vi "Update Values.vi"(8 "error in (no error)":errorcluster, 11 "TelemetryDebug in":refnum<class "TelemetryDebug.lvclass">) -> (0 "error out":errorcluster, 3 "TelemetryDebug out":refnum<class "TelemetryDebug.lvclass">)   [LabVIEW 2020, in "VectoTools.lvlib" / "TelemetryDebug.lvclass"]
uses:
  TelemetryDebug.lvclass
  Tree Entry.ctl
  TelemetryDebug.lvclass/TelemetryDebug.ctl
  Vecto/Group/Group.lvclass/Group.ctl
  Vecto/Group/Group.lvclass
  Vecto/DiscoveryService/DiscoveryService.lvclass
  Vecto/ChannelService/ChannelService.lvclass
  Vecto/Group Config/Group Config.lvclass
  Vecto/Channel Config/Channel Config.lvclass
panel:
  in  "Numeric":dbl format="%<%Y-%m-%dT%H:%M:%S%3u\n>T"
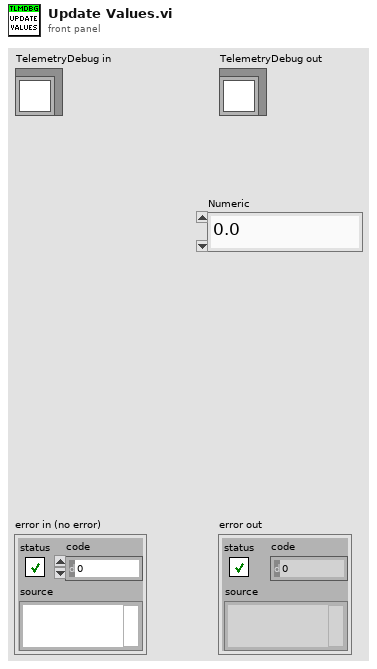
[diagram p1: front panel]
types:
  T1 = typedef "VectoTools.lvlib/TelemetryDebug.lvclass/Tree Entry.ctl" = cluster{"Hierarchy":string[], "Name":string, "Columns":string[]}
  T2 = typedef "Discovery.lvlib/Data.ctl" = cluster{"node_id":u32, "name":string, "ip":u32, "status":string, "services":T3[], "capabilities":string[], "system":string, "cluster":string, "app_version":string, "cfg_version":string}
  T3 = typedef "Service.lvlib/Data.ctl" = cluster{"type":T4, "port":i32}
  T4 = typedef "ServiceType.lvlib/Enumeration.ctl" = enum16{"SERVICETYPE_UNKNOWN", "SERVICETYPE_TCPSERVER", "SERVICETYPE_HTTPSERVER"}
  T5 = typedef "LVNodeAndColumnTypeDef.ctl" = cluster{"Node":string, "Column":i32}
  T6 = typedef "VectoConfig.lvlib/Group Info.ctl" = cluster{"System":string, "Cluster":string, "Node":string, "Task":string, "Name":string}
  T7 = typedef "VectoConfig.lvlib/Channel Info.ctl" = cluster{"Name":string, "Group":string, "Owning Node":string, "Owning Task":string, "Resource":string}
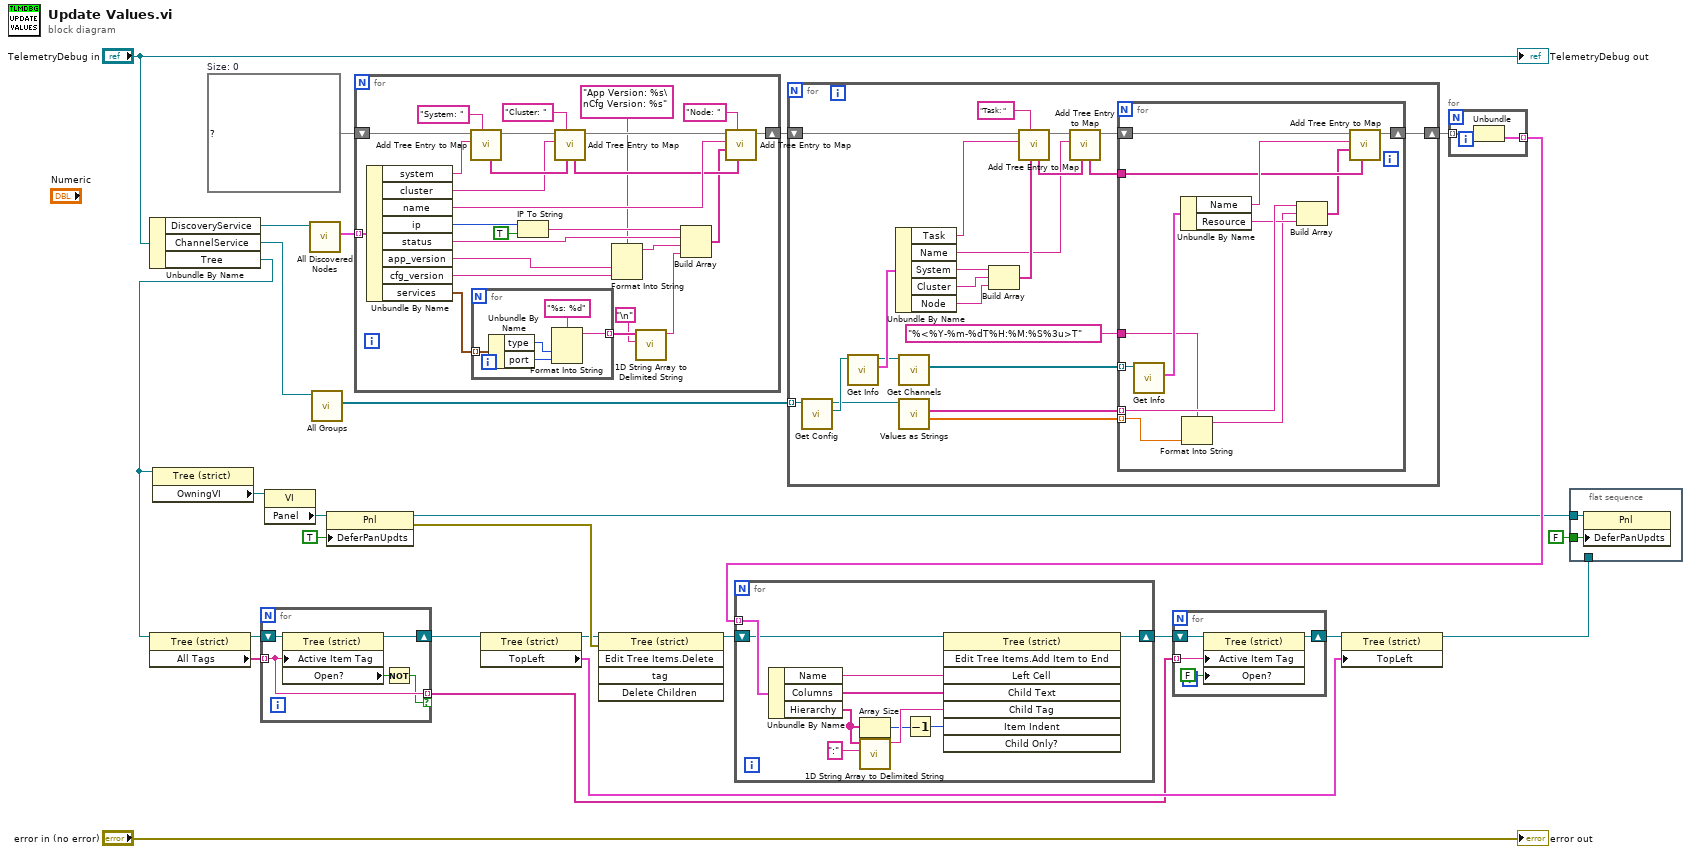
[diagram p0: block diagram]
diagram:
  w22 = map{string[], T1} {}  # Size: 0
  n1 = Unbundle By Name("TelemetryDebug in") -> ("DiscoveryService"=w24:refnum<class "DiscoveryService.lvclass">, "ChannelService"=w14:refnum<class "ChannelService.lvclass">, "Tree"=w1:refnum<vi>)
  n2 = property class="Tree (strict)"(reference=w1) -> (reference out=w7:refnum<vi>, "All Tags"=w8:string[])  [unwired: 1 in, 1 out]
  n3 = property class="Tree (strict)"(reference=w1) -> ("OwningVI"=w19:refnum<vi>)  [unwired: 1 in, 2 out]
  n4 = for {
    tunnel: w8 -> [w30] mode=indexing
    shift-right: [w28] -> w6
    shift-left: w7 -> [w32]
    tunnel: [w30] -> w5 mode=indexing if=w29
    n5 = property class="Tree (strict)"(reference=w32, "Active Item Tag"=w30) -> (reference out=w28:refnum<vi>, "Open?"=w31:bool)  [unwired: 1 in, 1 out]
    n6 = Not(x=w31) -> (.not. x?=w29:bool)
  }
  n7 = property class="VI"(reference=w19) -> ("Panel"=w18:refnum<vi>)  [unwired: 1 in, 2 out]
  n8 = call "All Discovered Nodes.vi"("DiscoveryService in"=w24) -> ("Nodes"=w23:T2[])  [unwired: 8 in, 2 out]
  n9 = call "All Groups.vi"("ChannelService in"=w14) -> ("Groups"=w11:refnum<class "Group.lvclass">[])  [unwired: 8 in, 2 out]
  n10 = property class="Pnl"(reference=w18, "DeferPanUpdts"=TRUE ("Defer Panel Updates")) -> (reference out=w15:refnum<vi>, error out=w27:errorcluster)  [unwired: 1 in]
  n11 = for {
    tunnel: w23 -> [w58] mode=indexing
    shift-right: [w49] -> w13
    shift-left: w22 -> [w57]
    n12 = Unbundle By Name(w58) -> ("system"=w56:string, "cluster"=w53:string, "name"=w51:string, "ip"=w48:u32, "status"=w44:string, "app_version"=w36:string, "cfg_version"=w35:string, "services"=w46:T3[])
    n13 = call "Add Tree Entry to Map.vi"("Name Prefix (none)"="System: ", "Name"=w56, "Map in"=w57) -> ("Map"=w54:map{string[], T1}, "Hierarchy"=w55:string[])  [unwired: 7 in]
    n14 = for {
      tunnel: w46 -> [w63] mode=indexing
      tunnel: [w59] -> w39 mode=indexing
      n15 = Unbundle By Name(w63) -> ("type"=w61:T4, "port"=w60:i32)
      n16 = Format Into String(format string="%s: %d", w61, w60) -> (resulting string=w59:string)  [unwired: 2 in, 1 out]
    }
    n17 = IP To String(1:TRUE ("dot notation? (F)"), 2:w48) -> (0:w45:string)
    n18 = call "Add Tree Entry to Map.vi"("Parent (None)"=w55, "Name Prefix (none)"="Cluster: ", "Name"=w53, "Map in"=w54) -> ("Map"=w52:map{string[], T1}, "Hierarchy"=w50:string[])  [unwired: 6 in]
    n19 = Format Into String(format string="App Version: %s\nCfg Version: %s", w36, w35) -> (resulting string=w33:string)  [unwired: 2 in, 1 out]
    n20 = call <vilib>:"1D String Array to Delimited String.vi"("delimiter"="\n", "string array"=w39) -> ("delimited string"=w38:string)  [unwired: 9 in]
    n21 = Build Array(w45, w44, w33, w38) -> (w43:string[])
    n22 = call "Add Tree Entry to Map.vi"("Parent (None)"=w50, "Name Prefix (none)"="Node: ", "Columns"=w43, "Name"=w51, "Map in"=w52) -> ("Map"=w49:map{string[], T1})  [unwired: 5 in, 1 out]
  }
  n23 = property class="Tree (strict)"(reference=w6) -> (reference out=w10:refnum<vi>, "TopLeft"=w9:T5)  [unwired: 1 in, 1 out]
  n24 = invoke class="Tree (strict)" method="Edit Tree Items.Delete"(reference=w10, error in=w27) -> (reference out=w20:refnum<vi>)  [unwired: 3 in, 4 out]
  n25 = for {
    shift-right: [w72] -> w12
    shift-left: w13 -> [w85]
    tunnel: w11 -> [w84] mode=indexing
    n26 = call "Get Config.vi"("Group in"=w84) -> ("Config"=w83:refnum<class "Group Config.lvclass">, "Group out"=w68:refnum<class "Group.lvclass">)  [unwired: 8 in, 1 out]
    n27 = call "Get Info.vi"("Group Config in"=w83) -> ("Info"=w82:T6, "Group Config out"=w70:refnum<class "Group Config.lvclass">)  [unwired: 8 in, 1 out]
    n28 = Unbundle By Name(w82) -> ("Task"=w77:string, "Name"=w74:string, "System"=w81:string, "Cluster"=w80:string, "Node"=w79:string)
    n29 = call "Get Channels.vi"("Group Config in"=w70) -> ("Channels"=w69:refnum<class "Channel Config.lvclass">[])  [unwired: 8 in, 2 out]
    n30 = call "Values as Strings.vi"("Group in"=w68) -> ("Timestamps"=w65:dbl[], "Value Strings"=w67:string[])  [unwired: 7 in, 2 out]
    n31 = Build Array(w81, w80, w79) -> (w78:string[])
    n32 = call "Add Tree Entry to Map.vi"("Parent (None)"=w78, "Name Prefix (none)"="Task: ", "Name"=w77, "Map in"=w85) -> ("Map"=w76:map{string[], T1}, "Hierarchy"=w75:string[])  [unwired: 6 in]
    n33 = call "Add Tree Entry to Map.vi"("Parent (None)"=w75, "Name"=w74, "Map in"=w76) -> ("Map"=w73:map{string[], T1}, "Hierarchy"=w71:string[])  [unwired: 7 in]
    n34 = for {
      shift-right: [w94] -> w72
      shift-left: w73 -> [w95]
      tunnel: w71 -> [w96]
      tunnel: w67 -> [w90] mode=indexing
      tunnel: w69 -> [w92] mode=indexing
      tunnel: w65 -> [w87] mode=indexing
      tunnel: "%<%Y-%m-%dT%H:%M:%S%3u>T" ("format string") -> [w88]
      n35 = call "Get Info.vi"("Channel Config in"=w92) -> ("Info"=w91:T7)  [unwired: 8 in, 2 out]
      n36 = Unbundle By Name(w91) -> ("Name"=w97:string, "Resource"=w89:string)
      n37 = Format Into String(format string=w88, w87) -> (resulting string=w86:string)  [unwired: 2 in, 1 out]
      n38 = Build Array(w90, w86, w89) -> (w93:string[])
      n39 = call "Add Tree Entry to Map.vi"("Parent (None)"=w96, "Columns"=w93, "Name"=w97, "Map in"=w95) -> ("Map"=w94:map{string[], T1})  [unwired: 6 in, 1 out]
    }
  }
  n40 = for {
    tunnel: w12 -> [w99] mode=indexing
    tunnel: [w98] -> w21 mode=indexing
    n41 = Unbundle(w99) -> ("Tree Entry"=w98:T1)  [unwired: 1 out]
  }
  n42 = for {
    tunnel: w21 -> [w109] mode=indexing
    shift-right: [w100] -> w2
    shift-left: w20 -> [w108]
    n43 = Unbundle By Name(w109) -> ("Name"=w107:string, "Columns"=w106:string[], "Hierarchy"=w103:string[])
    n44 = Array Size(array=w103) -> (size(s)=w102:i32)
    n45 = call <vilib>:"1D String Array to Delimited String.vi"("delimiter"=":", "string array"=w103) -> ("delimited string"=w104:string)  [unwired: 9 in]
    n46 = Decrement(x=w102) -> (x-1=w101:i32)
    n47 = invoke class="Tree (strict)" method="Edit Tree Items.Add Item to End"(reference=w108, "Left Cell"=w107, "Child Text"=w106, "Child Tag"=w104, "Item Indent"=w101) -> (reference out=w100:refnum<vi>)  [unwired: 3 in, 7 out]
  }
  n48 = for {
    shift-right: [w112] -> w4
    shift-left: w2 -> [w113]
    tunnel: w5 -> [w110] mode=indexing
    n49 = property class="Tree (strict)"(reference=w113, "Active Item Tag"=w110, "Open?"=FALSE ("Active Item:Open?")) -> (reference out=w112:refnum<vi>)  [unwired: 1 in, 1 out]
  }
  n50 = property class="Tree (strict)"(reference=w4, "TopLeft"=w9) -> (reference out=w3:refnum<vi>)  [unwired: 1 in, 1 out]
  n51 = flat-sequence {
    tunnel: FALSE ("Defer Panel Updates") -> [w115]
    tunnel: w15 -> [w114]
    tunnel: w3 -> [_]
    frame #0 {
      n52 = property class="Pnl"(reference=w114, "DeferPanUpdts"=w115) -> ()  [unwired: 1 in, 2 out]
    }
  }
  "error out" <- "error in (no error)"
  "TelemetryDebug out" <- "TelemetryDebug in"
